vi "选中的行上色.vi"(6 "颜色":cluster{"未选中颜色盒":u32, "选中颜色盒":u32}={"未选中颜色盒"=16763272, "选中颜色盒"=12439011}, 8 "错误输入（无错误）":errorcluster, 9 "这次的行":i32, 10 "上次的行":i32, 11 "引用":refnum<vi>) -> (0 "错误输出":errorcluster, 3 "上次的行输出":i32)   [LabVIEW 2013]
uses:
  <vilib>/Utility/miscctls.llb/LVRowAndColumnTypeDef.ctl
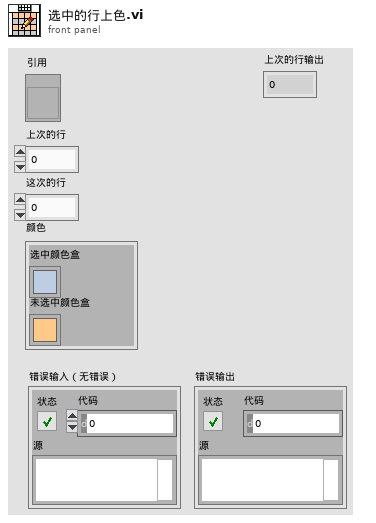
[diagram p1: front panel]
types:
  T1 = typedef "LVRowAndColumnTypeDef.ctl" = cluster{"Row":i32, "Column":i32}
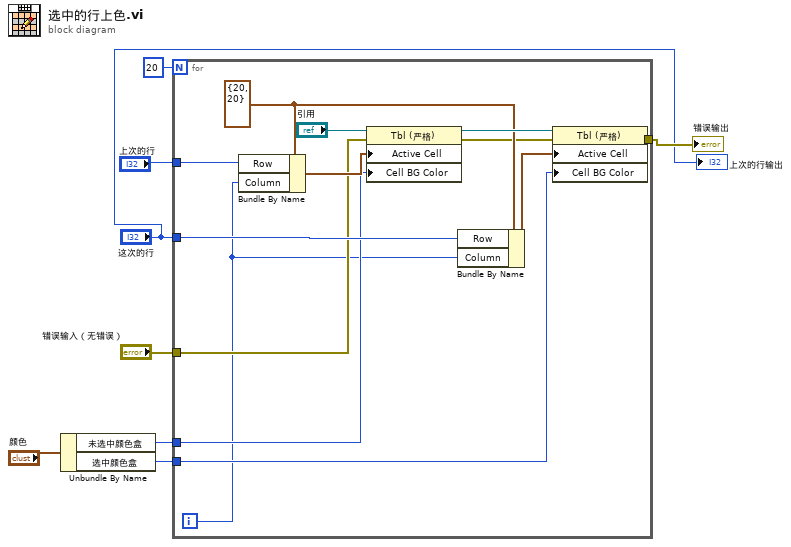
[diagram p0: block diagram]
diagram:
  n1 = Unbundle By Name("颜色") -> ("未选中颜色盒"=w6:u32, "选中颜色盒"=w5:u32)
  n2 = for {
    N: 20 -> [_]
    tunnel: "上次的行" -> [w19]
    tunnel: "这次的行" -> [w18]
    tunnel: w6 -> [w14]
    tunnel: w5 -> [w13]
    tunnel: "错误输入（无错误）" -> [w12]
    tunnel: [w10] -> w3
    i -> [w9]
    w17 = T1 {"Row"=20, "Column"=20} ("活动单元格:活动单元格")
    n3 = Bundle By Name(cluster=w17, "Row"=w19, "Column"=w9) -> (w15:T1)
    n4 = property on="属性节点" class="Tbl (严格)"(reference="引用", error in=w12, "Active Cell"=w15, "Cell BG Color"=w14) -> (reference out=w20:refnum<vi>, error out=w11:errorcluster)
    n5 = Bundle By Name(cluster=w17, "Row"=w18, "Column"=w9) -> (w16:T1)
    n6 = property on="属性节点" class="Tbl (严格)"(reference=w20, error in=w11, "Active Cell"=w16, "Cell BG Color"=w13) -> (error out=w10:errorcluster)  [unwired: 1 out]
  }
  "错误输出" <- w3
  "上次的行输出" <- "这次的行"
